vi "temp_collect_LT.vi"() -> (0 "counts":i32)   [LabVIEW 2013]
uses:
  phlib.dll
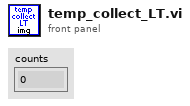
[diagram p1: front panel]
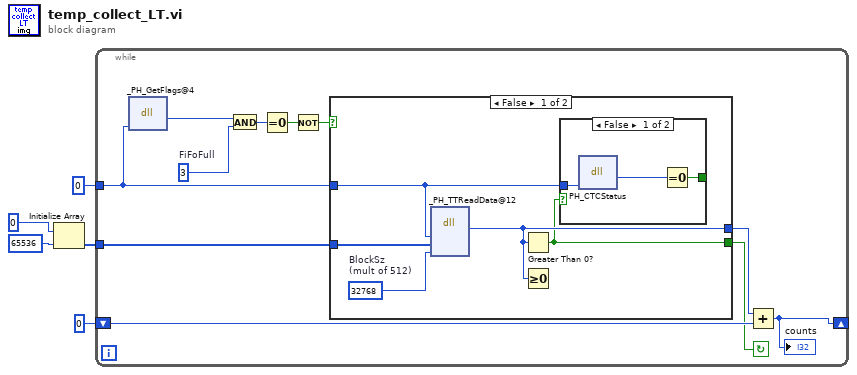
[diagram p0: block diagram]
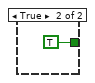
[diagram p2: hidden frame]
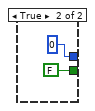
[diagram p3: hidden frame]
diagram:
  n1 = Initialize Array(u32 0, 65536) -> (w2:u32[])
  n2 = while {
    tunnel: 0 ("Deviceindex") -> [w11]
    tunnel: w2 -> [w10]
    shift-left: 0 -> [w16]
    shift-right: [w6] -> _
    stop <- w7 continue-if-true
    w12 = 3  # FiFoFull
    n3 = dll-call lib="phlib.dll" fn="_PH_GetFlags@4" label="PH_GetFlags"("devidx"=w11) -> (w14:i32)  [unwired: 4 in, 2 out]
    n4 = And(x=w14, y=w12) -> (x .and. y?=w13:i32)
    n5 = Equal To 0?(x=w13) -> (x = 0?=w15:bool)
    n6 = Not ("CTCDone")(x=w15) -> (.not. x?=w8:bool)
    n7 = case "In case of a FiFo overrun we must stop to avoid inconsistent data" shown="False" w8 {
      tunnel: w10 -> [w20 _]
      tunnel: [w21 0] -> w9
      tunnel: [w17 FALSE] -> w7
      tunnel: w11 -> [w18 _]
      frame False {
        w19 = 32768  # BlockSz (mult of 512)
        n8 = dll-call lib="phlib.dll" fn="_PH_TTReadData@12" label="PH_TTReadData"("devidx"=w18, "buffer"=w20, "blocksize"=w19) -> ("return type"=w21:i32)  [unwired: 6 in, 2 out]
        n9 = Greater Than 0?(x=w21) -> (x > 0?=w17:bool)
        n10 = Greater Or Equal To 0?(x=w21) -> ()  [unwired: 1 out]
        n11 = case shown="False" w17 {
          tunnel: [w23 TRUE] -> _
          tunnel: w18 -> [w22 _]
          frame False {
            n12 = dll-call lib="phlib.dll" fn="PH_CTCStatus"("devidx"=w22) -> (w24:i32)  [unwired: 4 in, 2 out]
            n13 = Equal To 0?(x=w24) -> (x = 0?=w23:bool)
          }
          frame True {
          }
        }
      }
      frame True {
      }
    }
    n14 = Add(x=w9, y=w16) -> (x+y=w6:i32)
    "counts" <- w6
  }
